vi "DDD Tdll.vi"(7 "dDdT":dbl, 8 "error in (no error)":errorcluster caption="错误输入（无错误）", 9 "x":dbl, 10 "d":dbl, 11 "t":dbl) -> (0 "error out":errorcluster caption="错误输出", 1 "x out":dbl, 2 "d out":dbl, 3 "t out":dbl, 5 "dDdT out":dbl)   [LabVIEW 2015]
doc: "void __cdecl DDDTdll(double *t, double *d, double *x, double *dDdT);"
uses:
  <userlib>/REFPROP/REFPROP.DLL
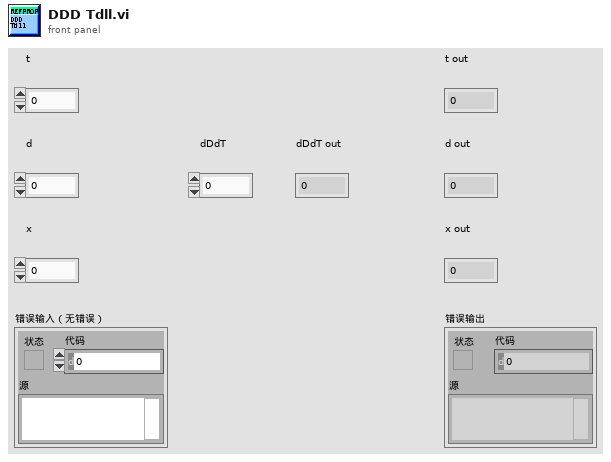
[diagram p1: front panel]
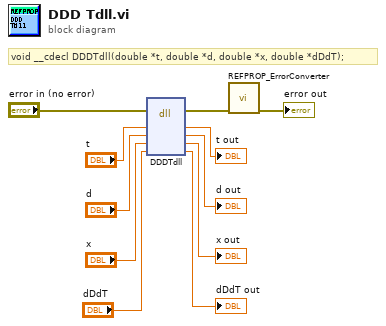
[diagram p0: block diagram]
diagram:
  # "void __cdecl DDDTdll(double *t, double *d, double *x, double *dDdT);"
  n1 = dll-call lib="C:/Program Files (x86)/National Instruments/LabVIEW 2015/user.lib/REFPROP/REFPROP.*" fn="DDDTdll"(error in="error in (no error)", "t"="t", "d"="d", "x"="x", "dDdT"="dDdT") -> (error out=w2:errorcluster, "t"=→"t out":dbl, "d"=→"d out":dbl, "x"=→"x out":dbl, "dDdT"=→"dDdT out":dbl)  [unwired: 3 in, 1 out]
  n2 = call <userlib>:"REFPROP_ErrorConverter.vi"("error in (no error)"=w2) -> ("error out"=→"error out":errorcluster)  [unwired: 10 in]
